vi "Exp02_GetAccAngle.vi"() -> ()   [LabVIEW 2019]
uses:
  <vilib>/myRIO/Instrument Drivers/Onboard IO/I2C/typedefs/I2C User Configuration.ctl
  <vilib>/myRIO/Instrument Drivers/Onboard IO/I2C/typedefs/I2C Transfer Rate.ctl
  <vilib>/Platform/TimedLoop/XDataNode/timing_clust.ctl
  <vilib>/Platform/TimedLoop/XDataNode/nitl_modes.ctl
  <vilib>/Platform/TimedLoop/XDataNode/wakeup.ctl
  <vilib>/Utility/error.llb/Error Cluster From Error Code.vi
  <vilib>/myRIO/Common/Instrument Driver Framework/myRIO v1.0/I2C/vis/myRIO v1.0 Configure I2C.vi
  <vilib>/myRIO/Common/Instrument Driver Framework/myRIO v1.0/I2C/vis/myRIO v1.0 Write I2C.vi
  <vilib>/myRIO/Common/Instrument Driver Framework/myRIO v1.0/I2C/vis/myRIO v1.0 Read I2C.vi
  <vilib>/Platform/TimedLoop/XDataNode/XDataNode.xnode
  <vilib>/myRIO/Instrument Drivers/Onboard IO/I2C/I2C.lvlib
  <vilib>/Platform/TimedLoop/XDataNode/XDNodeRunTimeDep.lvlib
panel:
  out "angle":dbl
  out "Bytes Read (decimal)":u8[](array[numeric]) format="%0d"
  out "Gyro Z":i16
  out "Gyro X":i16
  out "Gyro Y":i16
  out "Acc Z":i16
  out "Temperature":dbl
  out "Acc Y":i16
  out "Acc X":i16
  in  "stop":bool
  out "error out":errorcluster
  out "Bytes Read (binary)":u8[](array[numeric]) format="%08b"
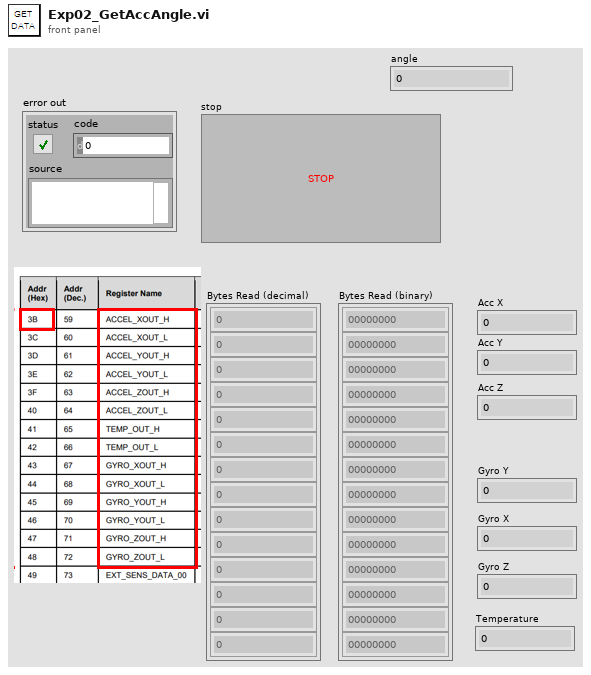
[diagram p1: front panel]
types:
  T1 = typedef "I2C.lvlib/I2C User Configuration.ctl" = cluster{"I2C Transfer Rate":T2}
  T2 = typedef "I2C.lvlib/I2C Transfer Rate.ctl" = enum16{"Standard mode (100 kbps)", "Fast mode (400 kbps)"}
  T3 = typedef "I2C.lvlib/I2C Reference.ctl" = cluster{"myRIO Reference":T4, "I2C Channels Enum":T8, "I2C Configuration":T9}
  T4 = typedef "myRIO Generic Hardware Reference.ctl" = cluster{"myRIO Model":T5, "myRIO Hardware Reference":T6}
  T5 = typedef "Hardware Version Enum.ctl" = enum16{"Unknown", "myRIO-1900", "myRIO-1950", "roboRIO", "NI ELVIS RIO CM", "ELVIS III"}
  T6 = typedef "myRIO v1.0 Reference.ctl" = cluster{"Generic FPGA Reference":T7, "Allow multiple opens":bool}
  T7 = typedef "Generic FPGA Reference.ctl" = refnum<k20>
  T8 = typedef "I2C Channels Enum.ctl" = enum16{"Not Connected", "A/I2C", "B/I2C", "I2C/I2C"}
  T9 = typedef "I2C.lvlib/I2C Configuration.ctl" = cluster{"I2C Transfer Rate":T2}
  T10 = typedef "XDNodeRunTimeDep.lvlib/timing_clust.ctl" = cluster{"Expected End [f-1]":u64, "Actual End [f-1]":u64, "Finished Late? [f-1]":bool, "Expected End [i-1]":u64, "Actual End [i-1]":u64, "Finished Late? [i-1]":bool, "Expected Start [i]":u64, "Actual Start [i]":u64, "Expected Start [f]":u64, "Actual Start [f]":u64, "Source Name":string, "Structure Name":string, "Period":i64, "Deadline":i64, "Offset":i64, "Start":i64, "Priority":i32, "Timeout":i32, "Mode":T11, "Wakeup Reason":T12, "Error":errorcluster, "Source Type":string, "Secondary Source Type":string, "Global End Time":u64, "Global Start Time":u64, "Frame Duration":u64, "Iteration Duration":u64, "Assigned CPU":i32, "I/O Scan Engine Mode":u32}
  T11 = typedef "XDNodeRunTimeDep.lvlib/nitl_modes.ctl" = enum32{"No Change", "Process missed periods, maintain original phase", "Discard missed periods, maintain original phase", "Process missed periods, ignore original phase", "Discard missed periods, ignore original phase"}
  T12 = typedef "XDNodeRunTimeDep.lvlib/wakeup.ctl" = enum32{"Normal", "Aborted", "Asynchronous wakeup", "Timing source error", "Timed loop error", "Timeout"}
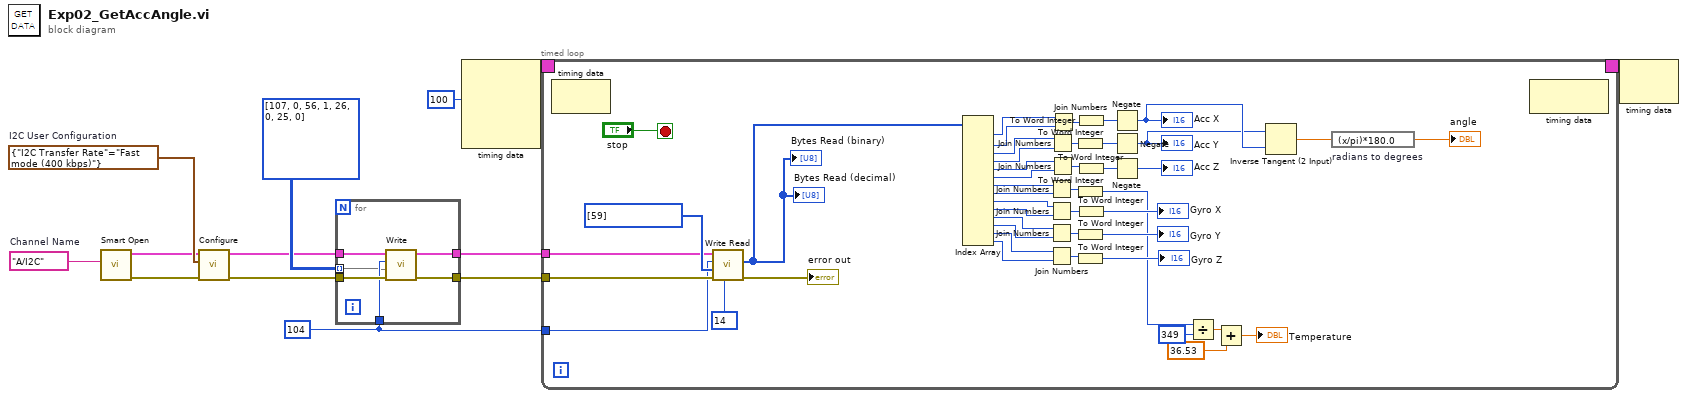
[diagram p0: block diagram]
diagram:
  w7 = u8 104 ("Slave Address (7-bit)")
  w12 = T1 {"I2C Transfer Rate"=enum."Fast mode (400 kbps)"}  # I2C User Configuration
  w13 = tag "A/I2C"  # Channel Name
  n1 = call <vilib>:"Smart Open.vi"("Channel Name"=w13) -> ("error out"=w10:errorcluster, "I2C Ref Out"=w11:T3)  [unwired: 9 in]
  n2 = call <vilib>:"Configure.vi"("error in (no error)"=w10, "I2C User Configuration"=w12, "I2C Ref In"=w11) -> ("error out"=w1:errorcluster, "I2C Ref Out"=w2:T3)  [unwired: 7 in]
  n3 = for {
    tunnel: w7 -> [w15]
    tunnel: w2 -> [w19]
    tunnel: [w16] -> w8
    tunnel: w1 -> [w18]
    tunnel: [w17] -> w9
    tunnel: u8[][] [[107, 0], [56, 1], [26, 0], [25, 0]] ("Bytes to Write") -> [w14] mode=indexing
    n4 = call <vilib>:"Write.vi"("error in (no error)"=w18, "Bytes to Write"=w14, "Slave Address (7-bit)"=w15, "I2C Ref In"=w19) -> ("error out"=w17:errorcluster, "I2C Ref Out"=w16:T3)  [unwired: 6 in]
  }
  n5 = node-c288(i64 100 ("Period")) -> (w6:T10)  [unwired: 3 in]
  n6 = timed-loop {
    timing: w6 -> [_]
    timing-out: [_] -> w5
    tunnel: w9 -> [w61]
    tunnel: w8 -> [w60]
    tunnel: w7 -> [w59]
    stop <- "stop" stop-if-true
    n7 = node-c288() -> ()  [unwired: 1 in, 1 out]
    n8 = call <vilib>:"Write Read.vi"("Byte Count"=u32 14, "error in (no error)"=w61, "Bytes to Write"=u8[] [59], "Slave Address (7-bit)"=w59, "I2C Ref In"=w60) -> ("error out"=→"error out":errorcluster, "Bytes Read"=w28:u8[])  [unwired: 3 in, 1 out]
    "Bytes Read (binary)" <- w28
    "Bytes Read (decimal)" <- w28
    n9 = Index Array(array=w28) -> (element #1=w57:u8, element #2=w56:u8, element #3=w55:u8, element #4=w54:u8, element #5=w53:u8, element #6=w52:u8, element #7=w51:u8, element #8=w50:u8, element #9=w49:u8, element #10=w48:u8, element #11=w47:u8, element #12=w46:u8, element #13=w45:u8, element #14=w44:u8)  [unwired: 14 in]
    n10 = Join Numbers(hi=w51, lo=w50) -> ((hi.lo)=w40:u16)
    n11 = Join Numbers(hi=w49, lo=w48) -> ((hi.lo)=w39:u16)
    n12 = Join Numbers(hi=w47, lo=w46) -> ((hi.lo)=w38:u16)
    n13 = Join Numbers(hi=w45, lo=w44) -> ((hi.lo)=w37:u16)
    n14 = Join Numbers(hi=w55, lo=w54) -> ((hi.lo)=w42:u16)
    n15 = Join Numbers(hi=w53, lo=w52) -> ((hi.lo)=w41:u16)
    n16 = Join Numbers(hi=w57, lo=w56) -> ((hi.lo)=w43:u16)
    n17 = To Word Integer(number=w42) -> (16bit integer=w23:i16)
    n18 = To Word Integer(number=w40) -> (16bit integer=w33:i16)
    n19 = To Word Integer(number=w38) -> (16bit integer=→"Gyro Y":i16)
    n20 = To Word Integer(number=w37) -> (16bit integer=→"Gyro Z":i16)
    n21 = To Word Integer(number=w43) -> (16bit integer=w25:i16)
    n22 = To Word Integer(number=w41) -> (16bit integer=w22:i16)
    n23 = To Word Integer(number=w39) -> (16bit integer=→"Gyro X":i16)
    n24 = Negate(x=w25) -> (-x=w24:i16)
    "Acc X" <- w24
    n25 = Negate(x=w23) -> (-x=w20:i16)
    "Acc Y" <- w20
    n26 = Negate(x=w22) -> (-x=→"Acc Z":i16)
    n27 = Divide(x=w33, y=i16 349) -> (x/y=w31:dbl)
    n28 = Add(x=w31, y=36.53) -> (x+y=→"Temperature":dbl)
    n29 = Inverse Tangent (2 Input)(1:w24, 2:w20) -> (0:w27:dbl)
    n30 = expression code="(x/pi)*180.0" "radians to degrees"(w27) -> (→"angle":dbl)
    n31 = node-c288() -> ()  [unwired: 1 in, 1 out]
  }
  n32 = node-c288(w5) -> ()  [unwired: 1 out]
